vi "CONV String to 1D Integer.vi"(0 "String":string, 1 "Delimiter (,)":string=",") -> (6 "1-D Integer":i32[](array[numeric]))   [LabVIEW 2017]
doc: "This routine converts a string list to a 1-D Integer array. String input may or may not have a trailing delimiter."
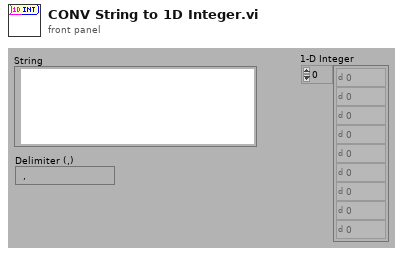
[diagram p1: front panel]
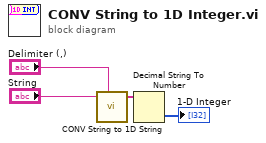
[diagram p0: block diagram]
diagram:
  n1 = call "CONV String to 1D String.vi"("String"="String", "Delimiter (,)"="Delimiter (,)") -> ("1-D String"=w1:string[])  [unwired: 7 out]
  n2 = Decimal String To Number(string=w1) -> (number=→"1-D Integer":i32[])  [unwired: 3 out]
